vi "Init.vi"(1 "Measurement Name":string, 2 "SA Pin":string, 3 "error in (no error)":errorcluster) -> (7 "CDMA2K_ACP out":refnum<class "CDMA2K_ACP.lvclass">, 10 "error out":errorcluster)   [LabVIEW 2016, in "SeqAuto Evaluations.lvlib" / "CDMA2K_ACP.lvclass"]
uses:
  CDMA2K_ACP.lvclass
  C:/Sequence Automation/Plugins/SeqAuto IEvaluation.lvlibp/SeqAuto IEvaluation.lvclass
  CDMA2K_ACP.lvclass/CDMA2K_ACP.ctl
  Plugins/SeqAuto IEvaluation.lvlibp/Write Measurement Name.vi
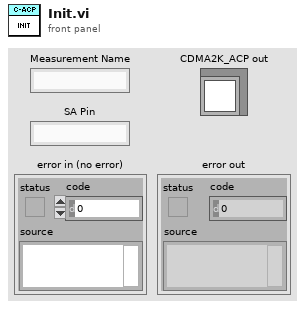
[diagram p1: front panel]
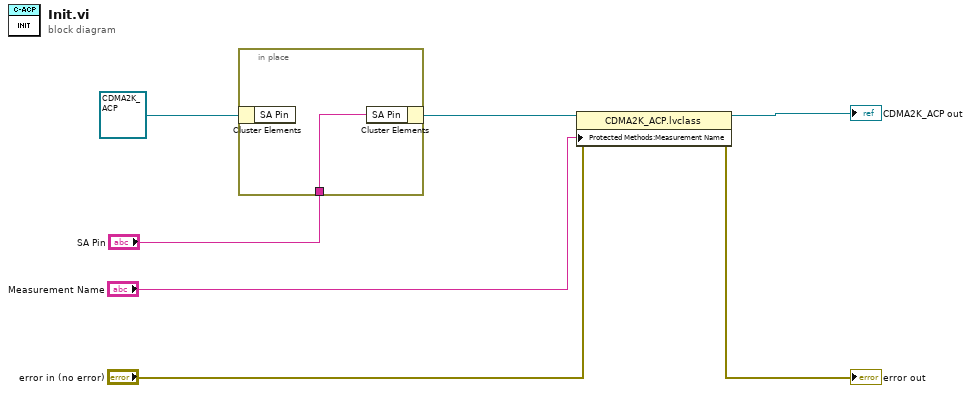
[diagram p0: block diagram]
diagram:
  n1 = in-place {
    in-place-border: "SA Pin" -> [w8]
    n2 = in-place-cluster #1(refnum<class "CDMA2K_ACP.lvclass"> refnum ("CDMA2K_ACP in")) -> ()  [unwired: 1 out]
    n3 = in-place-cluster #1("SA Pin"=w8) -> (w3:refnum<class "CDMA2K_ACP.lvclass">)
  }
  n4 = property class="CDMA2K_ACP.lvclass"(reference=w3, error in="error in (no error)", "Protected Methods:Measurement Name"="Measurement Name") -> (reference out=→"CDMA2K_ACP out":refnum<class "CDMA2K_ACP.lvclass">, error out=→"error out":errorcluster)
